vi "Filter_Table.vi"(11 "Table in":string[][](array[string])) -> (1 "2D":string[][](array[string]), 2 "Horizontal":string[][](array[string]), 3 "Vertical":string[][](array[string]))   [LabVIEW 2025]
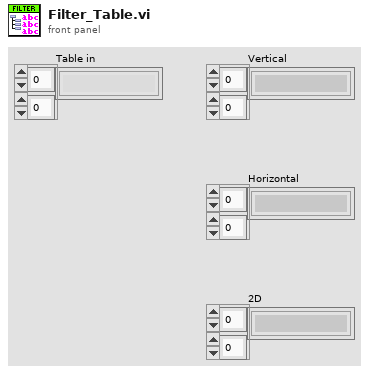
[diagram p1: front panel]
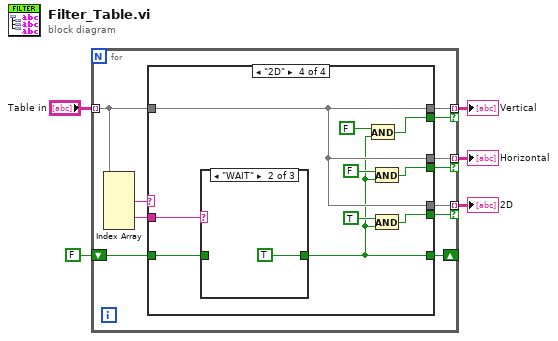
[diagram p0: block diagram]
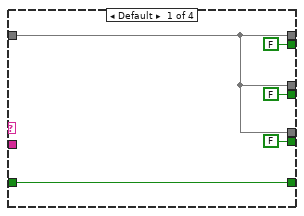
[diagram p2: hidden frame]
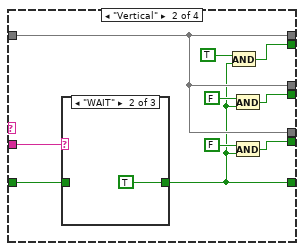
[diagram p3: hidden frame]
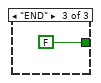
[diagram p5: hidden frame]
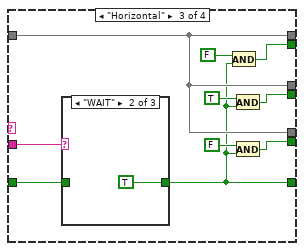
[diagram p6: hidden frame]
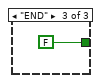
[diagram p8: hidden frame]
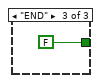
[diagram p10: hidden frame]
diagram:
  n1 = for {
    tunnel: "Table in" -> [w15] mode=indexing
    tunnel: [w14] -> w3 mode=indexing if=w11
    shift-right: [w12] -> _
    shift-left: FALSE -> [w13]
    tunnel: [w10] -> w4 mode=indexing if=w9
    tunnel: [w7] -> w5 mode=indexing if=w6
    n2 = Index Array(array=w15) -> (element #2=w16:string, element #4=w8:string)  [unwired: 5 in, 3 out]
    n3 = case shown="\"2D\"" w16 {
      tunnel: w15 -> [w18 w25 w38 w51]
      tunnel: [w18 w25 w38 w51] -> w14
      tunnel: w13 -> [w21 w30 w43 w56]
      tunnel: [w21 w22 w35 w48] -> w12
      tunnel: w8 -> [_ w31 w44 w57]
      tunnel: [FALSE w28 w41 w54] -> w11
      tunnel: [w18 w25 w38 w51] -> w10
      tunnel: [FALSE w26 w39 w52] -> w9
      tunnel: [w18 w25 w38 w51] -> w7
      tunnel: [FALSE w23 w36 w49] -> w6
      frame Default {
      }
      frame "Vertical" {
        n4 = case shown="\"WAIT\"" w31 {
          tunnel: [w32 TRUE FALSE] -> w22
          tunnel: w30 -> [w32 _ _]
          frame Default {
          }
          frame "WAIT" {
          }
          frame "END" {
          }
        }
        n5 = And(x=TRUE, y=w22) -> (x .and. y?=w28:bool)
        n6 = And(x=FALSE, y=w22) -> (x .and. y?=w26:bool)
        n7 = And(x=FALSE, y=w22) -> (x .and. y?=w23:bool)
      }
      frame "Horizontal" {
        n8 = case shown="\"WAIT\"" w44 {
          tunnel: [w45 TRUE FALSE] -> w35
          tunnel: w43 -> [w45 _ _]
          frame Default {
          }
          frame "WAIT" {
          }
          frame "END" {
          }
        }
        n9 = And(x=FALSE, y=w35) -> (x .and. y?=w41:bool)
        n10 = And(x=TRUE, y=w35) -> (x .and. y?=w39:bool)
        n11 = And(x=FALSE, y=w35) -> (x .and. y?=w36:bool)
      }
      frame "2D" {
        n12 = case shown="\"WAIT\"" w57 {
          tunnel: [w58 TRUE FALSE] -> w48
          tunnel: w56 -> [w58 _ _]
          frame Default {
          }
          frame "WAIT" {
          }
          frame "END" {
          }
        }
        n13 = And(x=FALSE, y=w48) -> (x .and. y?=w54:bool)
        n14 = And(x=FALSE, y=w48) -> (x .and. y?=w52:bool)
        n15 = And(x=TRUE, y=w48) -> (x .and. y?=w49:bool)
      }
    }
  }
  "Vertical" <- w3
  "Horizontal" <- w4
  "2D" <- w5
